vi "Para Model.vi"(10 "Table":string[][](array[string]), 11 "SW Config":T1) -> (3 "输出数组":string[][](array[string]))   [LabVIEW 2017]
uses:
  Ctrls/SW Config All.ctl
  Ctrls/SW Config Info.ctl
  Ctrls/SW Config Para.ctl
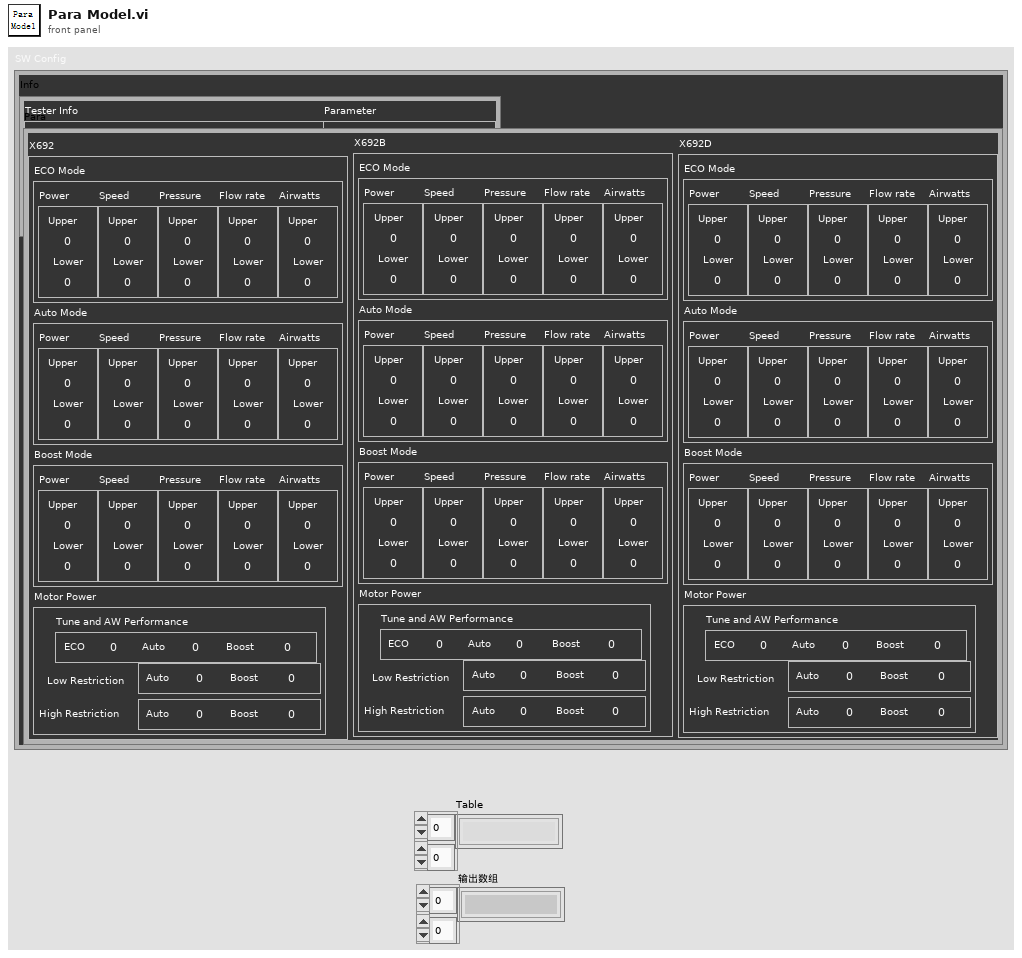
[diagram p1: front panel]
types:
  T1 = typedef "SW Config All.ctl" = cluster{"Info":T2, "Para":T3}
  T2 = typedef "SW Config Info.ctl" = cluster{"Tester Info":cluster{"EquipmentID":string, "Project  Name":string, "Tester ID":string, "ES NO.":string}, "Parameter":cluster{"UUT Type":string, "Product Mode":bool, " EVT1":bool, "Verify Tester":bool}}
  T3 = typedef "SW Config Para.ctl" = cluster{"X692":cluster{"ECO Mode":cluster{"Power":cluster{"Upper":dbl, "Lower":dbl}, "Speed":cluster{"Upper":dbl, "Lower":dbl}, "Pressure":cluster{"Upper":dbl, "Lower":dbl}, "Flow rate":cluster{"Upper":dbl, "Lower":dbl}, "Airwatts":cluster{"Upper":dbl, "Lower":dbl}}, "Auto Mode":cluster{"Power":cluster{"Upper":dbl, "Lower":dbl}, "Speed":cluster{"Upper":dbl, "Lower":dbl}, "Pressure":cluster{"Upper":dbl, "Lower":dbl}, "Flow rate":cluster{"Upper":dbl, "Lower":dbl}, "Airwatts":cluster{"Upper":dbl, "Lower":dbl}}, "Boost Mode":cluster{"Power":cluster{"Upper":dbl, "Lower":dbl}, "Speed":cluster{"Upper":dbl, "Lower":dbl}, "Pressure":cluster{"Upper":dbl, "Lower":dbl}, "Flow rate":cluster{"Upper":dbl, "Lower":dbl}, "Airwatts":cluster{"Upper":dbl, "Lower":dbl}}, "Motor Power":cluster{"Tune and AW Performance":cluster{"ECO":dbl, "Auto":dbl, "Boost ":dbl}, "Low Restriction":cluster{"Auto":dbl, "Boost ":dbl}, "High Restriction ":cluster{"Auto":dbl, "Boost ":dbl}}}, "X692B":cluster{"ECO Mode":cluster{"Power":cluster{"Upper":dbl, "Lower":dbl}, "Speed":cluster{"Upper":dbl, "Lower":dbl}, "Pressure":cluster{"Upper":dbl, "Lower":dbl}, "Flow rate":cluster{"Upper":dbl, "Lower":dbl}, "Airwatts":cluster{"Upper":dbl, "Lower":dbl}}, "Auto Mode":cluster{"Power":cluster{"Upper":dbl, "Lower":dbl}, "Speed":cluster{"Upper":dbl, "Lower":dbl}, "Pressure":cluster{"Upper":dbl, "Lower":dbl}, "Flow rate":cluster{"Upper":dbl, "Lower":dbl}, "Airwatts":cluster{"Upper":dbl, "Lower":dbl}}, "Boost Mode":cluster{"Power":cluster{"Upper":dbl, "Lower":dbl}, "Speed":cluster{"Upper":dbl, "Lower":dbl}, "Pressure":cluster{"Upper":dbl, "Lower":dbl}, "Flow rate":cluster{"Upper":dbl, "Lower":dbl}, "Airwatts":cluster{"Upper":dbl, "Lower":dbl}}, "Motor Power":cluster{"Tune and AW Performance":cluster{"ECO":dbl, "Auto":dbl, "Boost ":dbl}, "Low Restriction":cluster{"Auto":dbl, "Boost ":dbl}, "High Restriction ":cluster{"Auto":dbl, "Boost ":dbl}}}, "X692D":cluster{"ECO Mode":cluster{"Power":cluster{"Upper":dbl, "Lower":dbl}, "Speed":cluster{"Upper":dbl, "Lower":dbl}, "Pressure":cluster{"Upper":dbl, "Lower":dbl}, "Flow rate":cluster{"Upper":dbl, "Lower":dbl}, "Airwatts":cluster{"Upper":dbl, "Lower":dbl}}, "Auto Mode":cluster{"Power":cluster{"Upper":dbl, "Lower":dbl}, "Speed":cluster{"Upper":dbl, "Lower":dbl}, "Pressure":cluster{"Upper":dbl, "Lower":dbl}, "Flow rate":cluster{"Upper":dbl, "Lower":dbl}, "Airwatts":cluster{"Upper":dbl, "Lower":dbl}}, "Boost Mode":cluster{"Power":cluster{"Upper":dbl, "Lower":dbl}, "Speed":cluster{"Upper":dbl, "Lower":dbl}, "Pressure":cluster{"Upper":dbl, "Lower":dbl}, "Flow rate":cluster{"Upper":dbl, "Lower":dbl}, "Airwatts":cluster{"Upper":dbl, "Lower":dbl}}, "Motor Power":cluster{"Tune and AW Performance":cluster{"ECO":dbl, "Auto":dbl, "Boost ":dbl}, "Low Restriction":cluster{"Auto":dbl, "Boost ":dbl}, "High Restriction ":cluster{"Auto":dbl, "Boost ":dbl}}}}
  T4 = cluster{"ECO Mode":cluster{"Power":cluster{"Upper":dbl, "Lower":dbl}, "Speed":cluster{"Upper":dbl, "Lower":dbl}, "Pressure":cluster{"Upper":dbl, "Lower":dbl}, "Flow rate":cluster{"Upper":dbl, "Lower":dbl}, "Airwatts":cluster{"Upper":dbl, "Lower":dbl}}, "Auto Mode":cluster{"Power":cluster{"Upper":dbl, "Lower":dbl}, "Speed":cluster{"Upper":dbl, "Lower":dbl}, "Pressure":cluster{"Upper":dbl, "Lower":dbl}, "Flow rate":cluster{"Upper":dbl, "Lower":dbl}, "Airwatts":cluster{"Upper":dbl, "Lower":dbl}}, "Boost Mode":cluster{"Power":cluster{"Upper":dbl, "Lower":dbl}, "Speed":cluster{"Upper":dbl, "Lower":dbl}, "Pressure":cluster{"Upper":dbl, "Lower":dbl}, "Flow rate":cluster{"Upper":dbl, "Lower":dbl}, "Airwatts":cluster{"Upper":dbl, "Lower":dbl}}, "Motor Power":cluster{"Tune and AW Performance":cluster{"ECO":dbl, "Auto":dbl, "Boost ":dbl}, "Low Restriction":cluster{"Auto":dbl, "Boost ":dbl}, "High Restriction ":cluster{"Auto":dbl, "Boost ":dbl}}}
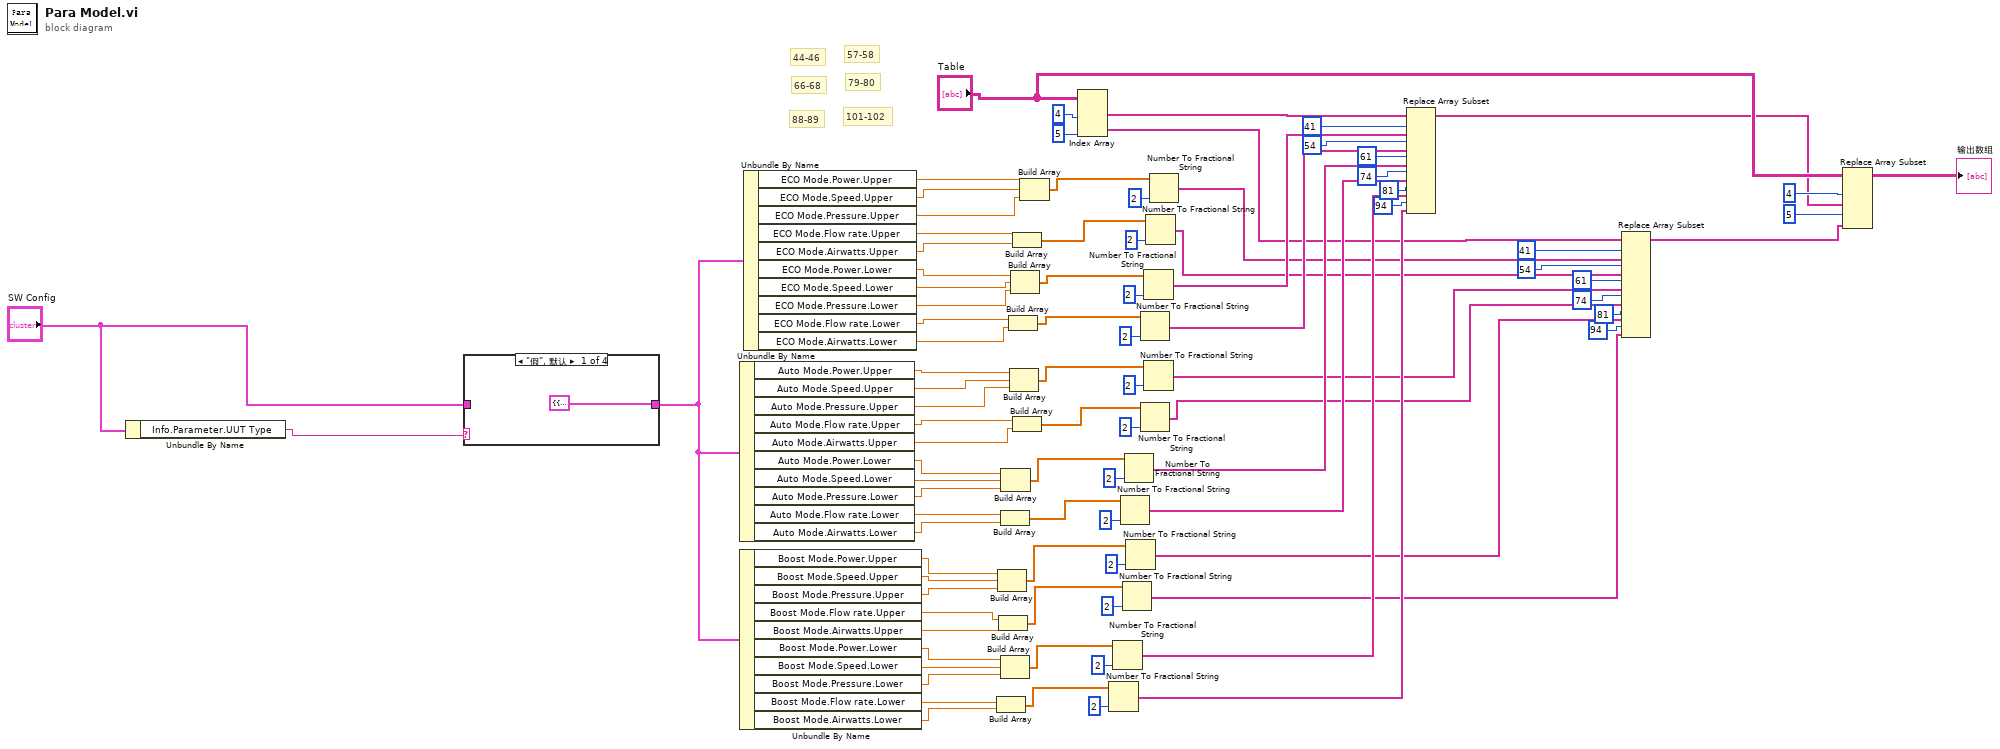
[diagram p0: block diagram]
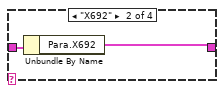
[diagram p2: hidden frame]
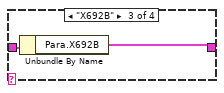
[diagram p3: hidden frame]
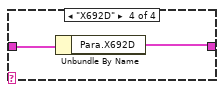
[diagram p4: hidden frame]
diagram:
  # "101-102"
  # "88-89"
  # "79-80"
  # "66-68"
  # "57-58"
  # "44-46"
  n1 = Unbundle By Name("SW Config") -> ("Info.Parameter.UUT Type"=w1:string)
  n2 = case shown="\"假\", 默认" w1 {
    tunnel: "SW Config" -> [_ w94 w96 w98]
    tunnel: [T4 {"ECO Mode"={"Power"={"Upper"=0.0, "Lower"=0.0}, "Speed"={"Upper"=0.0, "Lower"=0.0}, "Pressure"={"Upper"=0.0, "Lower"=0.0}, "Flow rate"={"Upper"=0.0, "Lower"=0.0}, "Airwatts"={"Upper"=0.0, "Lower"=0.0}}, "Auto Mode"={"Power"={"Upper"=0.0, "Lower"=0.0}, "Speed"={"Upper"=0.0, "Lower"=0.0}, "Pressure"={"Upper"=0.0, "Lower"=0.0}, "Flow rate"={"Upper"=0.0, "Lower"=0.0}, "Airwatts"={"Upper"=0.0, "Lower"=0.0}}, "Boost Mode"={"Power"={"Upper"=0.0, "Lower"=0.0}, "Speed"={"Upper"=0.0, "Lower"=0.0}, "Pressure"={"Upper"=0.0, "Lower"=0.0}, "Flow rate"={"Upper"=0.0, "Lower"=0.0}, "Airwatts"={"Upper"=0.0, "Lower"=0.0}}, "Motor Power"={"Tune and AW Performance"={"ECO"=0.0, "Auto"=0.0, "Boost "=0.0}, "Low Restriction"={"Auto"=0.0, "Boost "=0.0}, "High Restriction "={"Auto"=0.0, "Boost "=0.0}}} ("X692D") w93 w95 w97] -> w91
    frame "假", Default {
    }
    frame "X692" {
      n3 = Unbundle By Name(w94) -> ("Para.X692"=w93:T4)
    }
    frame "X692B" {
      n4 = Unbundle By Name(w96) -> ("Para.X692B"=w95:T4)
    }
    frame "X692D" {
      n5 = Unbundle By Name(w98) -> ("Para.X692D"=w97:T4)
    }
  }
  n6 = Unbundle By Name(w91) -> ("Auto Mode.Power.Upper"=w84:dbl, "Auto Mode.Speed.Upper"=w83:dbl, "Auto Mode.Pressure.Upper"=w82:dbl, "Auto Mode.Flow rate.Upper"=w68:dbl, "Auto Mode.Airwatts.Upper"=w67:dbl, "Auto Mode.Power.Lower"=w81:dbl, "Auto Mode.Speed.Lower"=w80:dbl, "Auto Mode.Pressure.Lower"=w79:dbl, "Auto Mode.Flow rate.Lower"=w66:dbl, "Auto Mode.Airwatts.Lower"=w65:dbl)
  n7 = Unbundle By Name(w91) -> ("Boost Mode.Power.Upper"=w78:dbl, "Boost Mode.Speed.Upper"=w77:dbl, "Boost Mode.Pressure.Upper"=w76:dbl, "Boost Mode.Flow rate.Upper"=w64:dbl, "Boost Mode.Airwatts.Upper"=w63:dbl, "Boost Mode.Power.Lower"=w75:dbl, "Boost Mode.Speed.Lower"=w74:dbl, "Boost Mode.Pressure.Lower"=w73:dbl, "Boost Mode.Flow rate.Lower"=w62:dbl, "Boost Mode.Airwatts.Lower"=w61:dbl)
  n8 = Unbundle By Name(w91) -> ("ECO Mode.Power.Upper"=w90:dbl, "ECO Mode.Speed.Upper"=w89:dbl, "ECO Mode.Pressure.Upper"=w88:dbl, "ECO Mode.Flow rate.Upper"=w72:dbl, "ECO Mode.Airwatts.Upper"=w71:dbl, "ECO Mode.Power.Lower"=w87:dbl, "ECO Mode.Speed.Lower"=w86:dbl, "ECO Mode.Pressure.Lower"=w85:dbl, "ECO Mode.Flow rate.Lower"=w70:dbl, "ECO Mode.Airwatts.Lower"=w69:dbl)
  n9 = Build Array(w62, w61) -> (w39:dbl[])
  n10 = Build Array(w78, w77, w76) -> (w12:dbl[])
  n11 = Build Array(w64, w63) -> (w11:dbl[])
  n12 = Build Array(w66, w65) -> (w46:dbl[])
  n13 = Build Array(w75, w74, w73) -> (w38:dbl[])
  n14 = Build Array(w81, w80, w79) -> (w47:dbl[])
  n15 = Build Array(w70, w69) -> (w52:dbl[])
  n16 = Build Array(w84, w83, w82) -> (w18:dbl[])
  n17 = Build Array(w87, w86, w85) -> (w57:dbl[])
  n18 = Build Array(w72, w71) -> (w23:dbl[])
  n19 = Build Array(w68, w67) -> (w17:dbl[])
  n20 = Build Array(w90, w89, w88) -> (w24:dbl[])
  n21 = Index Array ("索引数组")(array="Table", index (col) #1=4 ("禁用的索引 (列)"), index (col) #2=5 ("索引 (列)")) -> (element #1=w58:string[], element #2=w27:string[])  [unwired: 2 in]
  n22 = Number To Fractional String(number=w39, precision (6)=i16 2 ("精度(6)")) -> (F-format string=w36:string[])  [unwired: 2 in]
  n23 = Number To Fractional String(number=w38, precision (6)=i16 2 ("精度(6)")) -> (F-format string=w37:string[])  [unwired: 2 in]
  n24 = Number To Fractional String(number=w46, precision (6)=i16 2 ("精度(6)")) -> (F-format string=w44:string[])  [unwired: 2 in]
  n25 = Number To Fractional String(number=w11, precision (6)=i16 2 ("精度(6)")) -> (F-format string=w9:string[])  [unwired: 2 in]
  n26 = Number To Fractional String(number=w47, precision (6)=i16 2 ("精度(6)")) -> (F-format string=w45:string[])  [unwired: 2 in]
  n27 = Number To Fractional String(number=w12, precision (6)=i16 2 ("精度(6)")) -> (F-format string=w10:string[])  [unwired: 2 in]
  n28 = Number To Fractional String(number=w52, precision (6)=i16 2 ("精度(6)")) -> (F-format string=w51:string[])  [unwired: 2 in]
  n29 = Number To Fractional String(number=w17, precision (6)=i16 2 ("精度(6)")) -> (F-format string=w15:string[])  [unwired: 2 in]
  n30 = Number To Fractional String(number=w57, precision (6)=i16 2 ("精度(6)")) -> (F-format string=w55:string[])  [unwired: 2 in]
  n31 = Number To Fractional String(number=w18, precision (6)=i16 2 ("精度(6)")) -> (F-format string=w16:string[])  [unwired: 2 in]
  n32 = Number To Fractional String(number=w23, precision (6)=i16 2 ("精度(6)")) -> (F-format string=w21:string[])  [unwired: 2 in]
  n33 = Number To Fractional String(number=w24, precision (6)=i16 2 ("精度(6)")) -> (F-format string=w22:string[])  [unwired: 2 in]
  n34 = Replace Array Subset(array=w58, new element #1=w55, index #1=41 ("索引"), new element #2=w51, index #2=54 ("索引"), new element #3=w45, index #3=61 ("索引"), new element #4=w44, index #4=74 ("索引"), new element #5=w37, index #5=81 ("索引"), new element #6=w36, index #6=94 ("索引")) -> (w6:string[])
  n35 = Replace Array Subset(array=w27, new element #1=w22, index #1=41 ("索引"), new element #2=w21, index #2=54 ("索引"), new element #3=w16, index #3=61 ("索引"), new element #4=w15, index #4=74 ("索引"), new element #5=w10, index #5=81 ("索引"), new element #6=w9, index #6=94 ("索引")) -> (w4:string[])
  n36 = Replace Array Subset(array="Table", new element #1=w6, index (col) #1=4 ("禁用的索引 (列)"), new element #2=w4, index (col) #2=5 ("禁用的索引 (列)")) -> (→"输出数组":string[][])  [unwired: 2 in]
